vi "RT_static force ctrl_KA.vi"() -> ()   [LabVIEW 2019]
uses:
  <vilib>/Platform/TimedLoop/XDataNode/timing_clust.ctl
  <vilib>/Platform/TimedLoop/XDataNode/nitl_modes.ctl
  <vilib>/Platform/TimedLoop/XDataNode/wakeup.ctl
  <vilib>/FPGAPlugInAG/myRIO-1900/niLvFpga_Open_myRIO-1900.vi
  <vilib>/rvi/interface/common/dynamic/niFpgaDynamicAddResources.vi
  <vilib>/Utility/error.llb/Error Cluster From Error Code.vi
  <vilib>/rvi/errors/niLvFpgaAdjustHostInterfaceError.vi
  <vilib>/FPGAPlugInAG/Dynamic/niLvFpga_Close_Dynamic.vi
  <vilib>/Platform/TimedLoop/XDataNode/XDataNode.xnode
  <vilib>/rvi/interface/nirviOpenFPGA/nirviOpenFPGA.xnode
  FPGA Bitfiles/studentchallenge_FPGATarget_FPGARADCWDAC3_YedoVmsa1Hg.lvbitx
  FPGA_2R_ADC_W_DAC.vi
  <vilib>/rvi/interface/nirviReadWriteControl/nirviReadWriteControl.xnode
  <vilib>/rvi/interface/nirviCloseFPGA/nirviCloseFPGA.xnode
  <vilib>/Platform/TimedLoop/XDataNode/XDNodeRunTimeDep.lvlib
  NiFpgaLv.dll
  <vilib>/rvi/interface/Simulation/niFpgaSimulationCallBeginRW.vi
panel:
  in  "PID ON?":bool
  out "load cell out":dbl(graph)
  in  "stop":bool
  out "Cap Probe [mm]":dbl=0.43435006179715263 format="%.4f"
  out "Current [A]":dbl=-0.00198361231060317 format="%.4f"
  in  "Des Force [N]":dbl=0.3 format="%.3f"
  in  "Zero Cap":bool
  out "Force Control Late":i16
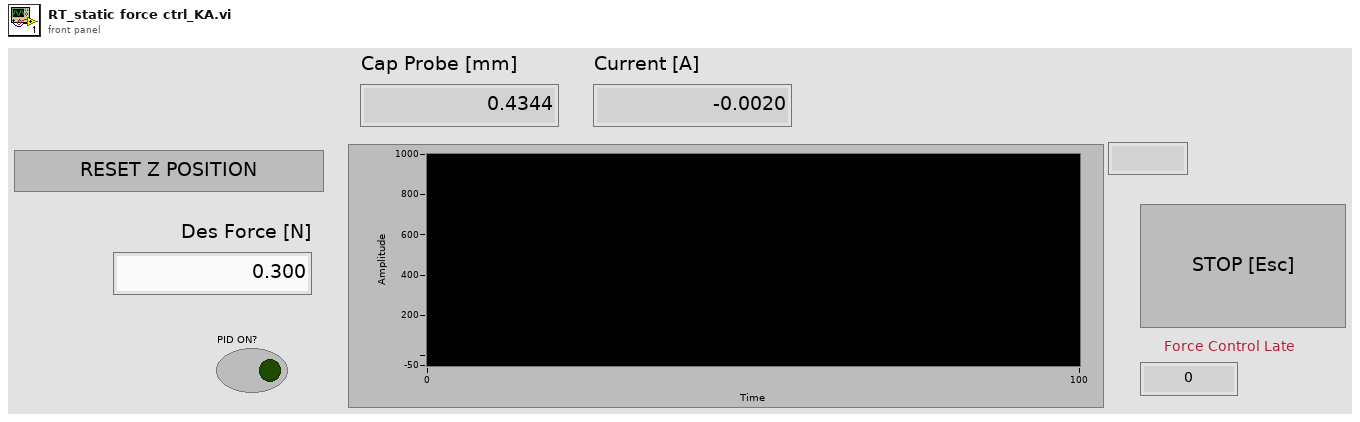
[diagram p1: front panel]
types:
  T1 = typedef "XDNodeRunTimeDep.lvlib/timing_clust.ctl" = cluster{"Expected End [f-1]":u64, "Actual End [f-1]":u64, "Finished Late? [f-1]":bool, "Expected End [i-1]":u64, "Actual End [i-1]":u64, "Finished Late? [i-1]":bool, "Expected Start [i]":u64, "Actual Start [i]":u64, "Expected Start [f]":u64, "Actual Start [f]":u64, "Source Name":string, "Structure Name":string, "Period":i64, "Deadline":i64, "Offset":i64, "Start":i64, "Priority":i32, "Timeout":i32, "Mode":T2, "Wakeup Reason":T3, "Error":errorcluster, "Source Type":string, "Secondary Source Type":string, "Global End Time":u64, "Global Start Time":u64, "Frame Duration":u64, "Iteration Duration":u64, "Assigned CPU":i32, "I/O Scan Engine Mode":u32}
  T2 = typedef "XDNodeRunTimeDep.lvlib/nitl_modes.ctl" = enum32{"No Change", "Process missed periods, maintain original phase", "Discard missed periods, maintain original phase", "Process missed periods, ignore original phase", "Discard missed periods, ignore original phase"}
  T3 = typedef "XDNodeRunTimeDep.lvlib/wakeup.ctl" = enum32{"Normal", "Aborted", "Asynchronous wakeup", "Timing source error", "Timed loop error", "Timeout"}
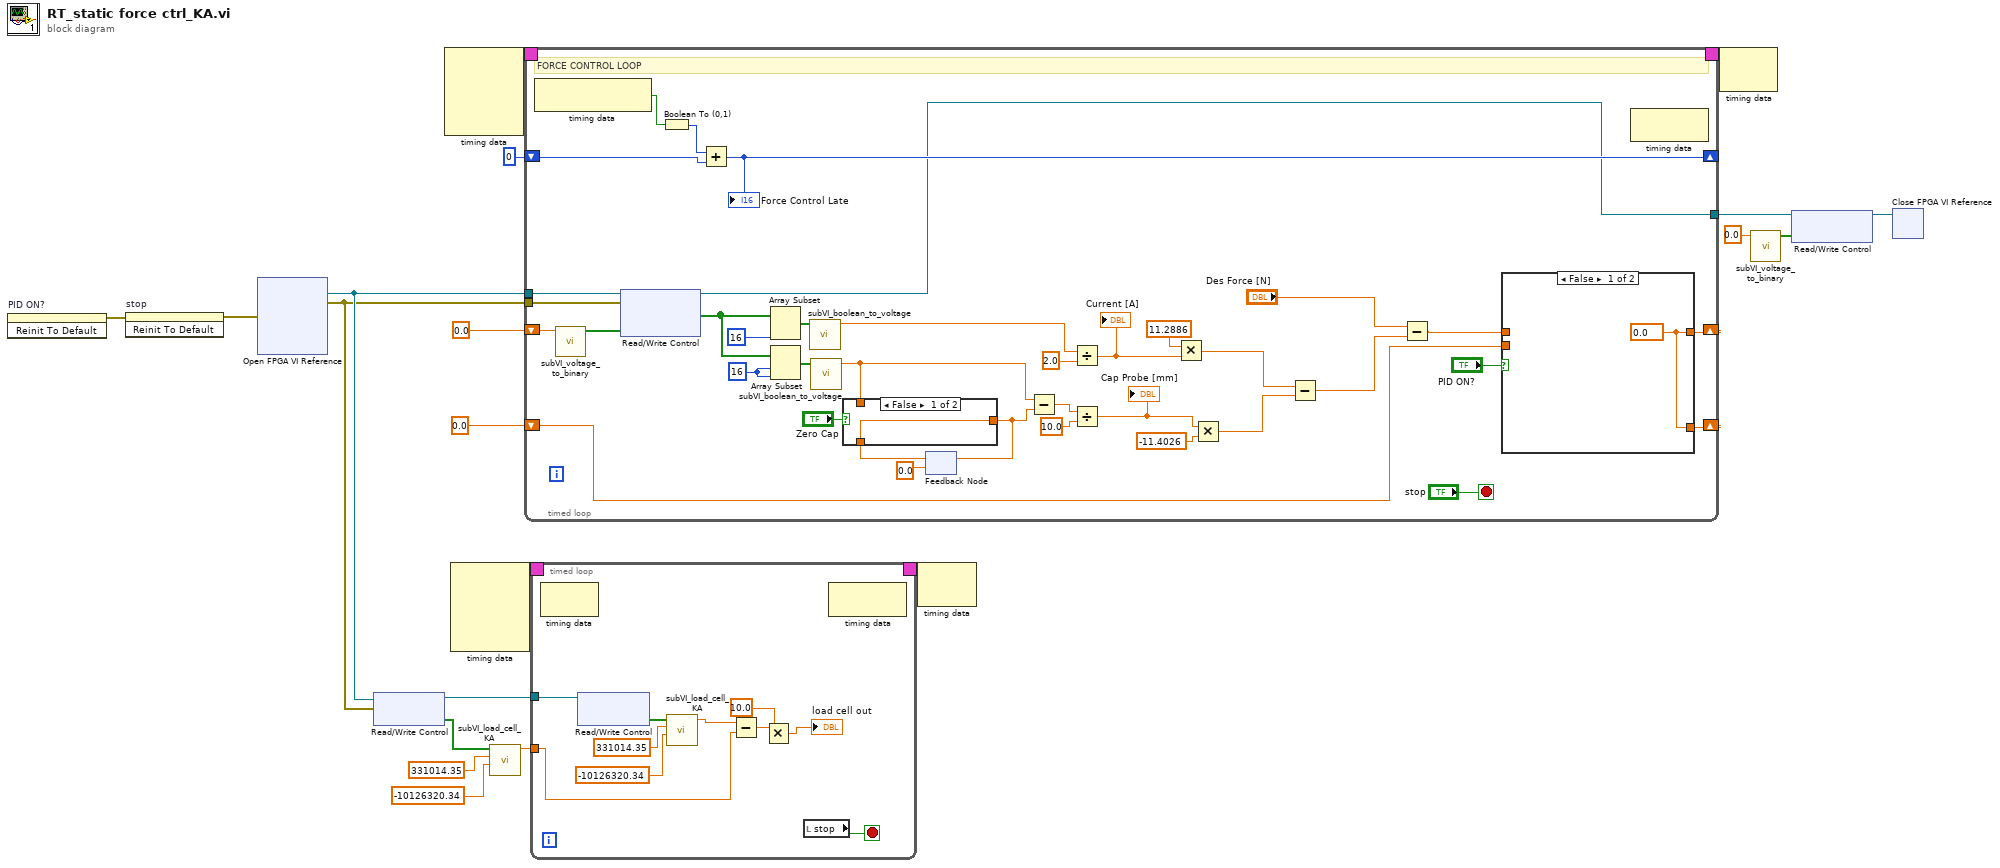
[diagram p0: block diagram]
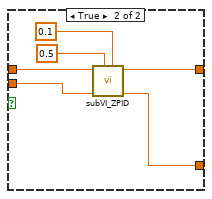
[diagram p2: hidden frame]
diagram:
  n1 = invoke on="PID ON?" class="Bool (strict)" method="Reinit To Default"() -> (error out=w1:errorcluster)  [unwired: 3 in, 2 out]
  n2 = invoke on="stop" class="Bool (strict)" method="Reinit To Default"(error in=w1) -> (error out=w8:errorcluster)  [unwired: 2 in, 2 out]
  n3 = xnode "Open FPGA VI Reference"("error in"=w8) -> ("FPGA VI Reference Out"=w7:refnum<k20>, "error out"=w6:errorcluster)  [unwired: 1 in]
  n4 = xnode "Read/Write Control"("FPGA VI Reference In"=w7, "error in"=w6) -> ("FPGA VI Reference Out"=w13:refnum<k20>, "Data array"=w12:bool[])  [unwired: 1 out]
  n5 = node-c288() -> (w20:T1)  [unwired: 4 in]
  n6 = node-c288() -> (w15:T1)  [unwired: 4 in]
  n7 = call "subVI_load_cell_KA.vi"("offset"=-10126320.34, "scale"=331014.35, "DATA ARRAY IN"=w12) -> ("LOAD OUT"=w9:dbl)  [unwired: 8 in]
  n8 = timed-loop {
    timing: w20 -> [_]
    timing-out: [_] -> w19
    tunnel: w7 -> [w40]
    tunnel: w6 -> [w39]
    shift-right: [w28] -> _
    shift-left: 0.0 -> [w36]
    shift-right: [w33] -> _
    shift-left: 0.0 ("Cumulative Error Out") -> [w23]
    shift-right: [w29] -> _
    shift-left: i16 0 -> [w32]
    tunnel: [w27] -> w5
    stop <- "stop" stop-if-true
    w56 = 16 ("length")
    # "FORCE CONTROL LOOP"
    n9 = node-c288() -> (w31:bool)  [unwired: 1 in]
    n10 = call "subVI_voltage_to_binary.vi"("voltage"=w36) -> ("binary"=w37:bool[])  [unwired: 10 in]
    n11 = xnode "Read/Write Control"("FPGA VI Reference In"=w40, "error in"=w39, "DAC 3 write"=w37) -> ("FPGA VI Reference Out"=w27:refnum<k20>, "ADC Read"=w49:bool[])  [unwired: 1 out]
    n12 = Boolean To (0,1)(Boolean=w31) -> (0, 1=w30:i16)
    n13 = Add(x=w30, y=w32) -> (x+y=w29:i16)
    "Force Control Late" <- w29
    n14 = Array Subset(array=w49, length=16) -> (w57:bool[])  [unwired: 1 in]
    n15 = Array Subset(array=w49, index=w56, length=w56) -> (w55:bool[])
    n16 = call "subVI_boolean_to_voltage.vi"("ADC read"=w57) -> ("V"=w34:dbl)  [unwired: 10 in]
    n17 = call "subVI_boolean_to_voltage.vi"("ADC read"=w55) -> ("V"=w43:dbl)  [unwired: 10 in]
    n18 = feedback #1(0.0) -> (w42:dbl)
    n19 = case shown="False" "Zero Cap" {
      tunnel: [w65 w66] -> w38
      tunnel: w42 -> [w65 _]
      tunnel: w43 -> [_ w66]
      frame False {
      }
      frame True {
      }
    }
    n20 = feedback-in #1(w38) -> ()
    n21 = Subtract(x=w43, y=w38) -> (x-y=w46:dbl)
    n22 = Divide(x=w34, y=2.0) -> (x/y=w50:dbl)
    "Current [A]" <- w50
    n23 = Divide(x=w46, y=10.0) -> (x/y=w41:dbl)
    "Cap Probe [mm]" <- w41
    n24 = Multiply(x=11.2886 ("BL"), y=w50) -> (x*y=w48:dbl)
    n25 = Multiply(x=w41, y=-11.4026 ("Stiffness [N/m]")) -> (x*y=w47:dbl)
    n26 = Subtract(x=w48, y=w47) -> (x-y=w25:dbl)
    n27 = Subtract(x="Des Force [N]", y=w25) -> (x-y=w24:dbl)
    n28 = case shown="False" "PID ON?" {
      tunnel: w24 -> [_ w64]
      tunnel: [w58 w63] -> w28
      tunnel: [w58 w60] -> w33
      tunnel: w23 -> [_ w59]
      frame False {
        w58 = 0.0 ("Z Manual")
      }
      frame True {
        n29 = call "subVI_ZPID.vi"("I"=0.1, "P"=0.5, "Cumulative Error In"=w59, "Error In"=w64) -> ("Cumulative Error Out"=w60:dbl, "Control Signal [V]"=w63:dbl)  [unwired: 6 in]
      }
    }
    n30 = node-c288() -> ()  [unwired: 1 in, 1 out]
  }
  n31 = timed-loop {
    timing: w15 -> [_]
    timing-out: [_] -> w14
    tunnel: w13 -> [w79]
    tunnel: w9 -> [w74]
    stop <- w70 stop-if-true
    n32 = node-c288() -> ()  [unwired: 1 in, 1 out]
    n33 = xnode "Read/Write Control"("FPGA VI Reference In"=w79) -> ("Data array"=w78:bool[])  [unwired: 1 in, 2 out]
    n34 = call "subVI_load_cell_KA.vi"("offset"=-10126320.34, "scale"=331014.35, "DATA ARRAY IN"=w78) -> ("LOAD OUT"=w75:dbl)  [unwired: 8 in]
    n35 = Subtract(x=w75, y=w74) -> (x-y=w73:dbl)
    n36 = Multiply(x=w73, y=10.0) -> (x*y=→"load cell out":dbl)
    n37 = local read "stop"() -> (w70:bool)
    n38 = node-c288() -> ()  [unwired: 1 in, 1 out]
  }
  n39 = node-c288(w14) -> ()  [unwired: 1 out]
  n40 = node-c288(w19) -> ()  [unwired: 1 out]
  n41 = call "subVI_voltage_to_binary.vi"("voltage"=0.0) -> ("binary"=w4:bool[])  [unwired: 10 in]
  n42 = xnode "Read/Write Control"("FPGA VI Reference In"=w5, "DAC 3 write"=w4) -> ("FPGA VI Reference Out"=w2:refnum<k20>)  [unwired: 1 in, 1 out]
  n43 = xnode "Close FPGA VI Reference"("FPGA VI Reference In"=w2) -> ()  [unwired: 1 in, 1 out]
